vi "Wait Until Not Busy on Specific Chip.vi"(6 "chip select  (1st chip)":enum16{"1st chip", "2nd chip"}(ring), 8 "error in (no error)":errorcluster, 11 "cluster of private data in":T1={"FPGA VI Reference"=refnum, "device index"=0, "screen size"=enum."8x1", "font size"=enum."5x8", "auto wrap"=FALSE, "alignment"=enum."None", "number of line"=enum."2 lines", "shift 0"=0, "entry mode 0"=enum."increment & no shift", "shift 1"=0, "entry mode 1"=enum."increment & no shift"}) -> (0 "error out":errorcluster, 3 "cluster of private data out":T1={"FPGA VI Reference"=refnum, "device index"=0, "screen size"=enum."8x1", "font size"=enum."5x8", "auto wrap"=FALSE, "alignment"=enum."None", "number of line"=enum."2 lines", "shift 0"=0, "entry mode 0"=enum."increment & no shift", "shift 1"=0, "entry mode 1"=enum."increment & no shift"})   [LabVIEW 2017, in "HD44780.lvclass"]
uses:
  HD44780.lvclass
  Common/HD44780 Common.lvlib
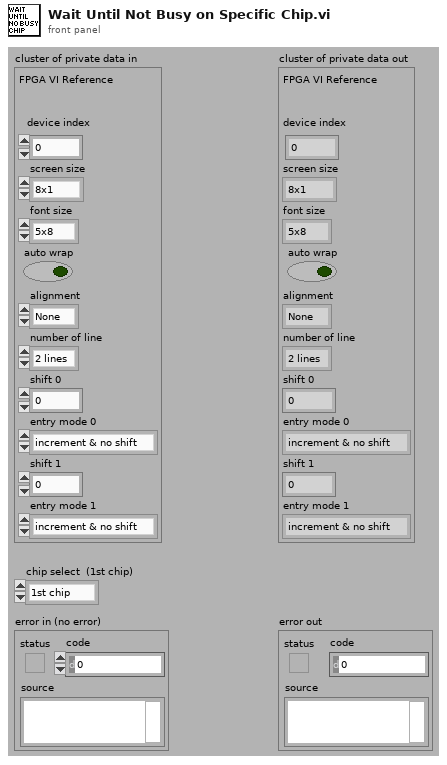
[diagram p1: front panel]
types:
  T1 = cluster{"FPGA VI Reference":refnum<k20>, "device index":i8, "screen size":enum8{"8x1", "8x2", "12x4", "16x1", "16x2", "16x4", "20x1", "20x2", "20x4", "24x1", "24x2", "40x2", "40x4"}, "font size":enum8{"5x8", "5x10"}, "auto wrap":bool, "alignment":enum16{"None", "Left", "Center", "Right"}, "number of line":enum8{"1 line", "2 lines"}, "shift 0":i8, "entry mode 0":enum8{"increment & no shift", "increment & shift", "decrement & no shift", "decrement & shift"}, "shift 1":i8, "entry mode 1":enum8{"increment & no shift", "increment & shift", "decrement & no shift", "decrement & shift"}}
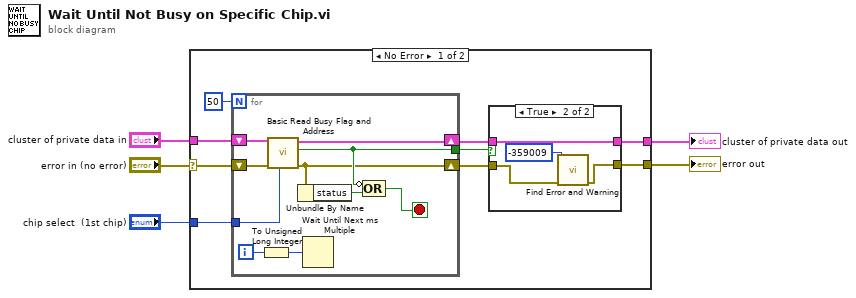
[diagram p0: block diagram]
diagram:
  n1 = case shown="No Error" "error in (no error)" {
    selector: "error in (no error)" -> [w7 w32]
    tunnel: [w12 w32] -> w4
    tunnel: [w9 w31] -> w3
    tunnel: "chip select  (1st chip)" -> [w8 _]
    tunnel: "cluster of private data in" -> [w6 w31]
    frame No Error {
      n2 = for {
        N: 50 -> [_]
        shift-right: [w23] -> w11
        shift-left: w7 -> [w29]
        tunnel: w8 -> [w28]
        tunnel: [w24] -> w13
        shift-right: [w22] -> w10
        shift-left: w6 -> [w21]
        i -> [w27]
        stop <- w25 stop-if-true
        n3 = To Unsigned Long Integer(number=w27) -> (unsigned 32bit integer=w26:u32)
        n4 = call "Basic Read Busy Flag and Address.vi"("chip select  (1st chip)"=w28, "error in (no error)"=w29, "cluster of private data in"=w21) -> ("error out"=w23:errorcluster, "busy flag"=w24:bool, "cluster of private data out"=w22:T1)  [unwired: 5 in, 1 out]
        n5 = Unbundle By Name(w23) -> ("status"=w30:bool)
        n6 = Wait Until Next ms Multiple(millisecond multiple=w26) -> ()  [unwired: 1 out]
        n7 = Compound Arithmetic op=OR(invert w24, w30) -> (w25:bool)
      }
      n8 = case shown="True" w13 {
        tunnel: [w15 w17] -> w12
        tunnel: w11 -> [w15 w18]
        tunnel: w10 -> [w16 w20]
        tunnel: [w16 w20] -> w9
        frame False {
        }
        frame True {
          n9 = call "Find Error and Warning.vi"("error in (no error)"=w18, "error code"=-359009) -> ("error out"=w17:errorcluster)  [unwired: 9 in]
        }
      }
    }
    frame Error {
    }
  }
  "error out" <- w4
  "cluster of private data out" <- w3
